vi "Get Active Numeric Function.vi"(0 "Numeric Functions in":refnum<class "Numeric Functions.lvclass">, 11 "error in (no error)":errorcluster) -> (4 "Numeric Functions out":refnum<class "Numeric Functions.lvclass">, 6 "Function":T1, 15 "error out":errorcluster)   [LabVIEW 2016, in "Numeric Functions.lvclass"]
uses:
  Numeric Functions.lvclass
  E:/Repository/LabVIEW Script Language/source code/LSL components/functions/functionsbase/functionbase.lvclass
  Function List.ctl
  functionsbase/functionbase.lvclass
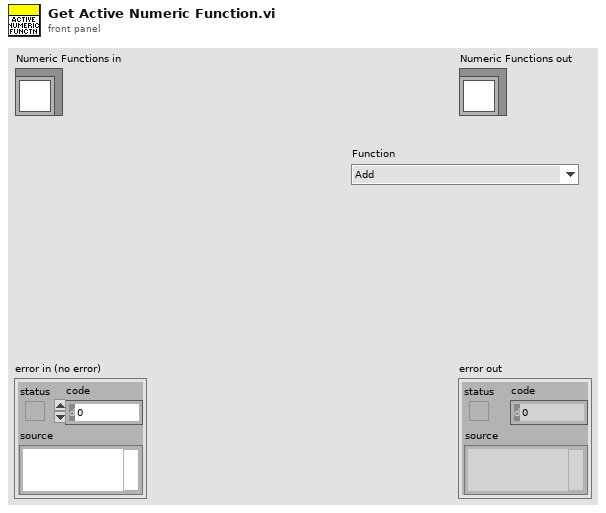
[diagram p1: front panel]
types:
  T1 = typedef "Numeric Functions.lvclass/Function List.ctl" = enum16{"Add", "Sub", "Multiply", "Divide", "Modulus", "Increament", "Decrement", "Square Root", "Square", "Negate", "Reciprocal", "Random Number"}
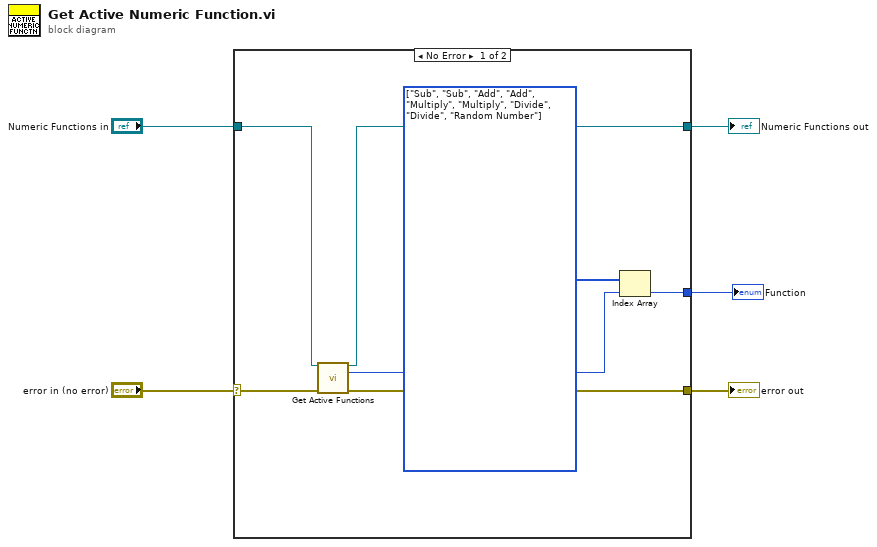
[diagram p0: block diagram]
diagram:
  n1 = case shown="No Error" "error in (no error)" {
    selector: "error in (no error)" -> [w10 w14]
    tunnel: [w8 w14] -> w4
    tunnel: [w7 w13] -> w2
    tunnel: "Numeric Functions in" -> [w9 w13]
    tunnel: [w11 _] -> w1
    frame No Error {
      w12 = T1[] [enum."Sub", enum."Sub", enum."Add", enum."Add", enum."Multiply", enum."Multiply", enum."Divide", enum."Divide", enum."Random Number"] items=["Add", "Sub", "Multiply", "Divide", "Modulus", "Increament", "Decrement", "Square Root", "Square", "Negate", "Reciprocal", "Random Number"]
      n2 = call "Get Active Functions.vi"("functionbase in"=w9, "error in (no error)"=w10) -> ("functionbase out"=w7:refnum<class "Numeric Functions.lvclass">, "Syntax Index"=w6:i32, "error out"=w8:errorcluster)  [unwired: 11 in]
      n3 = Index Array(array=w12, index=w6) -> (element=w11:T1)
    }
    frame Error {
    }
  }
  "error out" <- w4
  "Numeric Functions out" <- w2
  "Function" <- w1
